vi "Test.vi"() -> ()   [LabVIEW 2014, in "LVTiePie.lvlib"]
uses:
  LVTiePie.lvlib
panel:
  out "data value reference":refnum<data-value>
  out "VI Refnum":refnum<vi>
  out "initialized array":dbl[](array[numeric])
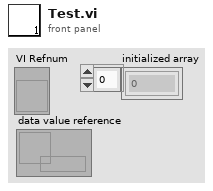
[diagram p1: front panel]
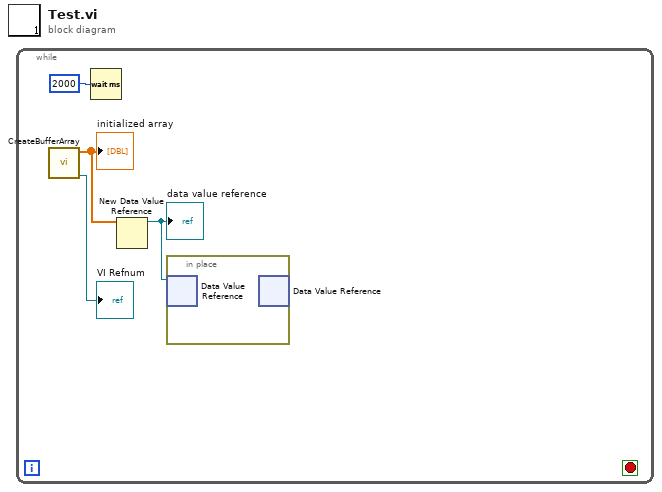
[diagram p0: block diagram]
diagram:
  n1 = while {
    stop <- _ stop-if-true
    n2 = call "CreateBufferArray.vi"() -> ("VI Refnum"=→"VI Refnum":refnum<vi>, "initialized array"=w2:dbl[])  [unwired: 10 in]
    "initialized array" <- w2
    n3 = Wait (ms)(milliseconds to wait=u32 2000) -> ()  [unwired: 1 out]
    n4 = New Data Value Reference(data value=w2) -> (data value reference=w1:refnum<data-value>)  [unwired: 1 in, 1 out]
    "data value reference" <- w1
    n5 = in-place {
      n6 = in-place-dvr #1(w1) -> ()  [unwired: 2 out]
      n7 = in-place-dvr #1() -> ()  [unwired: 1 in, 2 out]
    }
  }
